vi "DAQmx立即写数字端口.vi"() -> ()   [LabVIEW 2010]
uses:
  <vilib>/DAQmx/write.llb/DAQmx Write.vi
  <vilib>/DAQmx/write.llb/DAQmx Write (Digital Bool 1Line 1Point).vi
  <vilib>/daqmx/miscellaneous.llb/DAQmx Fill In Error Info.vi
panel:
  in  "data":bool
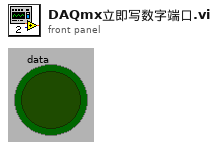
[diagram p1: front panel]
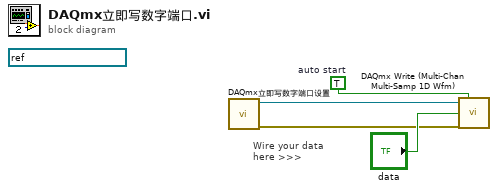
[diagram p0: block diagram]
diagram:
  (unwired) refnum<k21> "MyDigitalInTask"
  w4 = TRUE  # auto start
  # "Wire your data\nhere >>>"
  n1 = call "DAQmx立即写数字端口设置.vi"() -> ("error out"=w1:errorcluster, "task out"=w2:refnum<k21>)  [unwired: 10 in]
  n2 = call-poly "DAQmx Write (Multi-Chan Multi-Samp 1D Wfm).vi"("task/channels in"=w2, "auto start"=w4, "data"="data", "error in"=w1) -> ()  [unwired: 9 in, 3 out]
